vi "Data Storage - DRAM Arbiter.vi"(0 "# of empty slots available":u32, 1 "# of inputs available":u32, 2 "memory mode":bool, 3 "reset":bool, 5 "input write":bool, 7 "# of outputs ready for":u32, 9 "# of pending reads":u16, 11 "# of words available":u32, 12 "request for data":bool, 13 "burst length":u16, 14 "priority (balanced)":T1) -> (4 "write enable":bool, 6 "read enable":bool)   [LabVIEW 2018, in "Streaming FPGA.lvlib"]
doc: "DRAM Memory read/write arbiter for the Data Storage. In case the storage is used in FIFO mode (<B>memory mode</B> is false) this VI balances dynamically between the DRAM write and read accesses to maximize the throughput. In case the storage is used in Memory mode (<B>memory mode</B> is true) this VI enables only DRAM writes until the memory becomes full, then it enables only read operations.\n\nInputs:\n\n<B># of inputs available</B>: The number of elements the DRAM Memory writer can provide without blocking starting from the current cycle.\n\n<B># of empty slots available</B>: The number of elements available in the DRAM for writing.\n\n<B>input write</B>: Set this input to true if the DRAM is written in the current cycle.\n\n<B># of outputs ready for</B>: The number of elements the DRAM Memory reader can accept without blocking starting from the current cycle.\n\n<B># of pending reads</B>: The number of DRAM read requests pending.\n\n<B># of words available</B>: The number of elements available in the DRAM for reading (number of elements for which no read is requested yet).\n\n<B>request for data</B>: Set this input to true if data is requested from the DRAM in the current cycle.\n\n<B>memory mode</B>: A false on this input selects FIFO mode, a true selects Memory mode. In case of FIFO mode this VI balances dynamically between the DRAM write and read accesses to maximize the throughput. In case of Memory mode this VI enables only DRAM writes until the memory becomes full, then it enables only read operations.\n\n<B>burst length</B>: In case of FIFO mode this VI issues DRAM read and write requests in separate time periods. In each period this VI initiates either only read operations or only write operations to perform <B>burst length</B> number of (read or write) operations. When a period ends a decision is made what operations to perform in the next period.\n\n<B>priority</B>: Use this input to select which operations to favor in FIFO mode. The \"favor writes\" option gives priority to DRAM writes, the \"favor reads\" option gives priority to DRAM reads. The \"balanced\" option balances between DRAM reads and writes.\n\nOutputs:\n\n<B>write enable</B>: A true on this output indicates that the DRAM may be written in the next cycle. A false on this output indicates that the DRAM should not be written in the next cycle.\n\n<B>read enable</B>: A true on this output indicates that a read request may be issued to the DRAM in the next cycle. A false on this output indicates that a read request should not be issued to the DRAM in the next cycle."
uses:
  Streaming FPGA.lvlib
  Data Storage - DRAM FIFO Priority.ctl
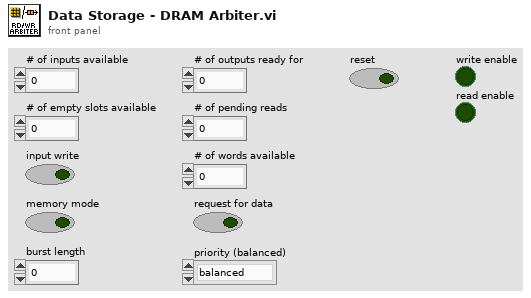
[diagram p1: front panel]
types:
  T1 = typedef "Streaming FPGA.lvlib/Data Storage - DRAM FIFO Priority.ctl" = enum16{"balanced", "favor writes", "favor reads"}
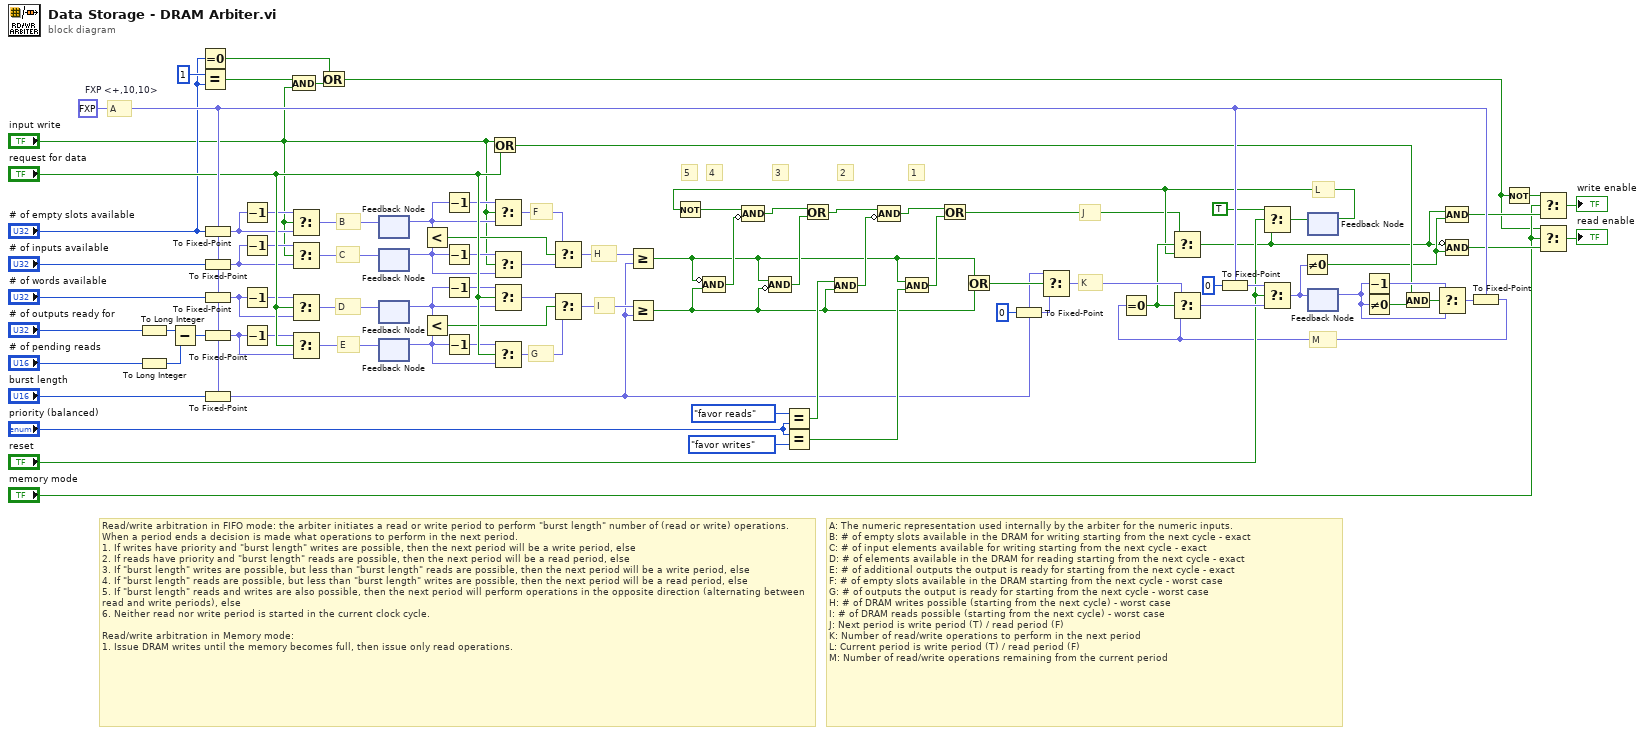
[diagram p0: block diagram]
diagram:
  w90 = fxp<+,10,10> 0.0  # FXP <+,10,10>
  # "1"
  # "2"
  # "3"
  # "4"
  # "5"
  # "G"
  # "E"
  # "F"
  # "B"
  # "I"
  # "H"
  # "K"
  # "J"
  # "Read/write arbitration in FIFO mode: the arbiter initiates a read or write period to perform \"burst length\" number of (read or write) operations. When a period ends a decision is made what operations to perform in the next period.\n1. If writes have priority and \"burst length\" writes are possible, then the next period will be a write period, else\n2. If reads have priority and \"burst length\" reads are possible, then the next period will be a read period, else\n3. If \"burst length\" writes are possible, but less than \"burst length\" reads are possible, then the next period will be a write period, else\n4. If \"burst length\" reads are possible, but less than \"burst length\" writes are possible, then the next period will be a read period, else\n5. If \"burst length\" reads and writes are also possible, then the next period will perform operations in the opposite direction (alternating between read and write periods), else\n6. Neither read nor write period is started in the current clock cycle.\n\nRead/write arbitration in Memory mode:\n1. Issue DRAM writes until the memory becomes full, then issue only read operations."
  # "A"
  # "M"
  # "L"
  # "D"
  # "C"
  # "A: The numeric representation used internally by the arbiter for the numeric inputs.\nB: # of empty slots available in the DRAM for writing starting from the next cycle - exact\nC: # of input elements available for writing starting from the next cycle - exact\nD: # of elements available in the DRAM for reading starting from the next cycle - exact\nE: # of additional outputs the output is ready for starting from the next cycle - exact\nF: # of empty slots available in the DRAM starting from the next cycle - worst case\nG: # of outputs the output is ready for starting from the next cycle - worst case\nH: # of DRAM writes possible (starting from the next cycle) - worst case\nI: # of DRAM reads possible (starting from the next cycle) - worst case\nJ: Next period is write period (T) / read period (F)\nK: Number of read/write operations to perform in the next period\nL: Current period is write period (T) / read period (F)\nM: Number of read/write operations remaining from the current period"
  n1 = To Long Integer(number="# of outputs ready for") -> (32bit integer=w58:i32)
  n2 = To Long Integer(number="# of pending reads") -> (32bit integer=w57:i32)
  n3 = Subtract(x=w58, y=w57) -> (x-y=w56:i32)
  n4 = Equal To 0?(x="# of empty slots available") -> (x = 0?=w3:bool)
  n5 = Equal?(x=u32 1, y="# of empty slots available") -> (x = y?=w6:bool)
  n6 = To Fixed-Point(fixed-point type=w90, number="# of empty slots available") -> (fixed-point=w67:fxp<+,10,10>)
  n7 = To Fixed-Point(fixed-point type=w90, number="# of inputs available") -> (fixed-point=w54:fxp<+,10,10>)
  n8 = To Fixed-Point(fixed-point type=w90, number="# of words available") -> (fixed-point=w55:fxp<+,10,10>)
  n9 = To Fixed-Point(fixed-point type=w90, number=w56) -> (fixed-point=w63:fxp<+,10,10>)
  n10 = To Fixed-Point(fixed-point type=w90, number="burst length") -> (fixed-point=w24:fxp<+,10,10>)
  n11 = Decrement(x=w67) -> (x-1=w75:fxp<+/-,11,11>)
  n12 = Decrement(x=w54) -> (x-1=w77:fxp<+/-,11,11>)
  n13 = Decrement(x=w55) -> (x-1=w76:fxp<+/-,11,11>)
  n14 = Decrement(x=w63) -> (x-1=w64:fxp<+/-,11,11>)
  n15 = And(x=w6, y="input write") -> (x .and. y?=w4:bool)
  n16 = Select(t=w75, s="input write", f=w67) -> (s? t:f=w73:fxp<+/-,11,11>)
  n17 = Select(t=w77, s="input write", f=w54) -> (s? t:f=w74:fxp<+/-,11,11>)
  n18 = Select(t=w76, s="request for data", f=w55) -> (s? t:f=w78:fxp<+/-,11,11>)
  n19 = Select(t=w64, s="request for data", f=w63) -> (s? t:f=w62:fxp<+/-,11,11>)
  n20 = Or(x=w3, y=w4) -> (x .or. y?=w2:bool)
  n21 = feedback #1() -> (w53:fxp<+/-,11,11>)  [unwired: 1 in]
  n22 = feedback-in #1(w73) -> ()
  n23 = feedback-in #2(w74) -> ()
  n24 = feedback #2() -> (w52:fxp<+/-,11,11>)  [unwired: 1 in]
  n25 = feedback #3() -> (w49:fxp<+/-,11,11>)  [unwired: 1 in]
  n26 = feedback-in #3(w78) -> ()
  n27 = feedback #4() -> (w48:fxp<+/-,11,11>)  [unwired: 1 in]
  n28 = feedback-in #4(w62) -> ()
  n29 = Less?(x=w53, y=w52) -> (x < y?=w50:bool)
  n30 = Less?(x=w49, y=w48) -> (x < y?=w46:bool)
  n31 = Decrement(x=w53) -> (x-1=w71:fxp<+/-,11,11>)
  n32 = Decrement(x=w52) -> (x-1=w72:fxp<+/-,11,11>)
  n33 = Decrement(x=w49) -> (x-1=w70:fxp<+/-,11,11>)
  n34 = Decrement(x=w48) -> (x-1=w61:fxp<+/-,11,11>)
  n35 = Or(x="input write", y="request for data") -> (x .or. y?=w18:bool)
  n36 = Select(t=w71, s="input write", f=w53) -> (s? t:f=w41:fxp<+/-,11,11>)
  n37 = Select(t=w72, s="input write", f=w52) -> (s? t:f=w51:fxp<+/-,11,11>)
  n38 = Select(t=w70, s="request for data", f=w49) -> (s? t:f=w47:fxp<+/-,11,11>)
  n39 = Select(t=w61, s="request for data", f=w48) -> (s? t:f=w42:fxp<+/-,11,11>)
  n40 = Select(t=w41, s=w50, f=w51) -> (s? t:f=w39:fxp<+/-,11,11>)
  n41 = Select(t=w47, s=w46, f=w42) -> (s? t:f=w40:fxp<+/-,11,11>)
  n42 = Greater Or Equal?(x=w39, y=w24) -> (x >= y?=w27:bool)
  n43 = Greater Or Equal?(x=w40, y=w24) -> (x >= y?=w26:bool)
  n44 = Compound Arithmetic op=AND(invert w27, w26) -> (w36:bool)
  n45 = Compound Arithmetic op=AND(w27, invert w26) -> (w34:bool)
  n46 = Equal?(x=Data_Storage_-_DRAM_FIFO_Priority."favor reads", y="priority (balanced)") -> (x = y?=w33:bool)
  n47 = Equal?(x="priority (balanced)", y=Data_Storage_-_DRAM_FIFO_Priority."favor writes") -> (x = y?=w30:bool)
  n48 = And(x=w33, y=w26) -> (x .and. y?=w32:bool)
  n49 = And(x=w27, y=w30) -> (x .and. y?=w28:bool)
  n50 = Or(x=w27, y=w26) -> (x .or. y?=w25:bool)
  n51 = To Fixed-Point(fixed-point type=w24, number=u8 0) -> (fixed-point=w23:fxp<+,10,10>)
  n52 = Select(t=w24, s=w25, f=w23) -> (s? t:f=w88:fxp<+,10,10>)
  n53 = To Fixed-Point(fixed-point type=w90, number=i16 0) -> (fixed-point=w82:fxp<+,10,10>)
  n54 = feedback #5() -> (w38:bool)  [unwired: 1 in]
  n55 = Not(x=w38) -> (.not. x?=w37:bool)
  n56 = Compound Arithmetic op=AND(w37, invert w36) -> (w35:bool)
  n57 = Or(x=w35, y=w34) -> (x .or. y?=w31:bool)
  n58 = Compound Arithmetic op=AND(w31, invert w32) -> (w29:bool)
  n59 = Or(x=w29, y=w28) -> (x .or. y?=w21:bool)
  n60 = feedback #6() -> (w20:fxp<+,10,10>)  [unwired: 1 in]
  n61 = Decrement(x=w20) -> (x-1=w69:fxp<+/-,11,11>)
  n62 = Not Equal To 0?(x=w20) -> (x != 0?=w19:bool)
  n63 = And(x=w18, y=w19) -> (x .and. y?=w17:bool)
  n64 = Select(t=w69, s=w17, f=w20) -> (s? t:f=w68:fxp<+/-,11,11>)
  n65 = To Fixed-Point(fixed-point type=w90, number=w68) -> (fixed-point=w66:fxp<+,10,10>)
  n66 = Equal To 0?(x=w66) -> (x = 0?=w85:bool)
  n67 = Select(t=w21, s=w85, f=w38) -> (s? t:f=w14:bool)
  n68 = Select(t=w88, s=w85, f=w66) -> (s? t:f=w87:fxp<+,10,10>)
  n69 = Select(t=TRUE, s="reset", f=w14) -> (s? t:f=w86:bool)
  n70 = Select(t=w82, s="reset", f=w87) -> (s? t:f=w16:fxp<+,10,10>)
  n71 = Not Equal To 0?(x=w16) -> (x != 0?=w15:bool)
  n72 = feedback-in #5(w86) -> ()
  n73 = feedback-in #6(w16) -> ()
  n74 = Compound Arithmetic op=AND(w14, w15) -> (w13:bool)
  n75 = Compound Arithmetic op=AND(invert w14, w15) -> (w11:bool)
  n76 = Not(x=w2) -> (.not. x?=w1:bool)
  n77 = Select(t=w1, s="memory mode", f=w13) -> (s? t:f=→"write enable":bool)
  n78 = Select(t=w2, s="memory mode", f=w11) -> (s? t:f=→"read enable":bool)
